vi "Array difference.vi"(2 "Array 2":cluster{"String":string, "String 2":string}[](array[cluster]), 3 "Array 1":cluster{"String":string, "String 2":string}[](array[cluster])) -> (0 "Array 2-(array1&2)":cluster{"String":string, "String 2":string}[](array[cluster]), 1 "Array 1-(array1&2)":cluster{"String":string, "String 2":string}[](array[cluster]))   [LabVIEW 2011]
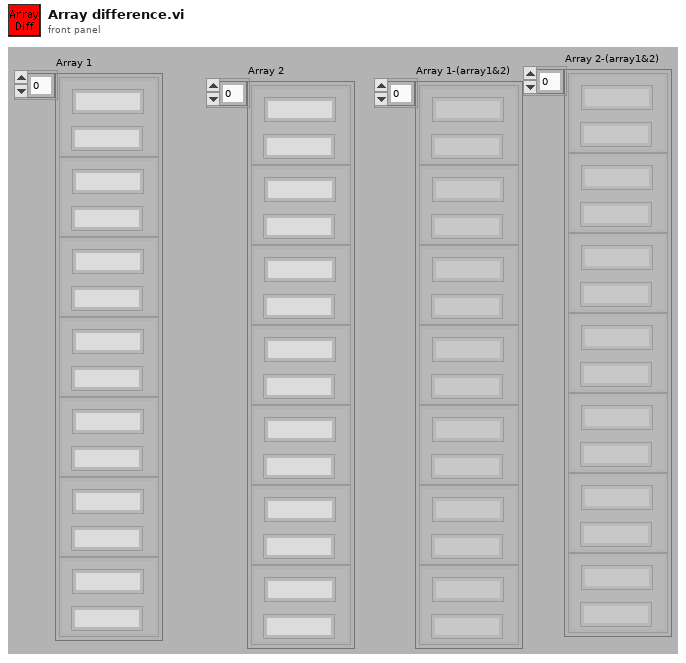
[diagram p1: front panel]
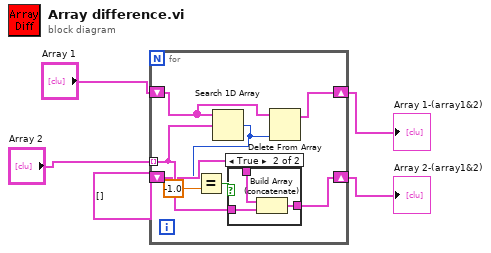
[diagram p0: block diagram]
diagram:
  n1 = for {
    tunnel: "Array 2" -> [w11] mode=indexing
    shift-right: [w12] -> w4
    shift-left: "Array 1" -> [w13]
    shift-right: [w10] -> w1
    shift-left: cluster{"String":string, "String 2":string}[] [] -> [w9]
    n2 = Search 1D Array(1D array=w13, element=w11) -> (index of element=w6:i32)  [unwired: 1 in]
    n3 = Equal?(x=w6, y=-1.0) -> (x = y?=w8:bool)
    n4 = case shown="True" w8 {
      tunnel: w11 -> [_ w17]
      tunnel: [w14 w16] -> w10
      tunnel: w9 -> [w14 w15]
      frame False {
      }
      frame True {
        n5 = Build Array (concatenate)(w15, w17) -> (w16:cluster{"String":string, "String 2":string}[])
      }
    }
    n6 = Delete From Array(array=w13, index=w6) -> (array with subset deleted=w12:cluster{"String":string, "String 2":string}[])  [unwired: 1 in, 1 out]
  }
  "Array 1-(array1&2)" <- w4
  "Array 2-(array1&2)" <- w1
